vi "callRsgui.vi"(11 "path":path=path "D:/vicomm case/CUB/17ce1/02272020/Radar - 2015 32bit_autoqueue_bigMotion") -> ()   [LabVIEW 2015]
panel:
  out "standard error":string
  out "standard output":string
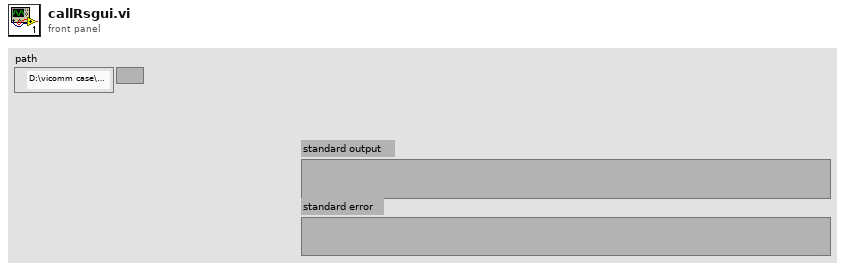
[diagram p1: front panel]
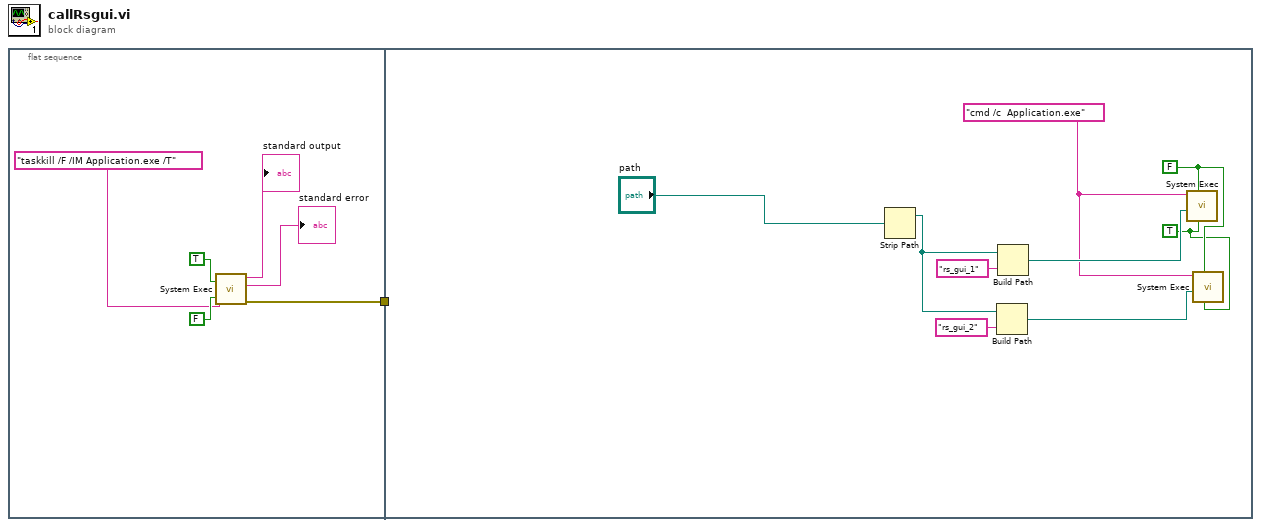
[diagram p0: block diagram]
diagram:
  n1 = flat-sequence {
    tunnel: [w4] -> w1
    tunnel: w1 -> [_]
    frame #0 {
      n2 = call <vilib>:"System Exec.vi"("run minimized? (F)"=FALSE, "wait until completion? (T)"=TRUE, "command line"="taskkill /F /IM Application.exe /T") -> ("error out"=w4:errorcluster, "standard error"=→"standard error":string, "standard output"=→"standard output":string)  [unwired: 5 in, 1 out]
    }
    frame #1 {
      w8 = TRUE ("run minimized? (F)")
      w9 = FALSE ("wait until completion? (T)")
      w10 = "cmd /c  Application.exe" ("command line")
      n3 = Strip Path(path="path") -> (stripped path=w13:path)  [unwired: 1 out]
      n4 = Build Path(base path=w13, name or relative path="rs_gui_2") -> (appended path=w11:path)
      n5 = Build Path(base path=w13, name or relative path="rs_gui_1") -> (appended path=w12:path)
      n6 = call <vilib>:"System Exec.vi"("run minimized? (F)"=w8, "wait until completion? (T)"=w9, "working directory"=w12, "command line"=w10) -> ()  [unwired: 4 in, 4 out]
      n7 = call <vilib>:"System Exec.vi"("run minimized? (F)"=w8, "wait until completion? (T)"=w9, "working directory"=w11, "command line"=w10) -> ()  [unwired: 4 in, 4 out]
    }
  }
